vi "Fire DAQAcqModeChanged Event_DAQ.vi"(8 "error in (no error)":errorcluster, 10 "DAQState":variant, 11 "DAQ_Engine in":refnum<class "DAQ_Engine.lvclass">) -> (0 "error out":errorcluster, 3 "DAQ_Engine out":refnum<class "DAQ_Engine.lvclass">)   [LabVIEW 2019, in "DAQ_Engine.lvclass"]
doc: "Developed by Kevin Thompson\nkevin@thompsonengineering.net\n\nCopyright 2018-2020\nThompson Engineering, LLC"
uses:
  DAQ_Engine.lvclass
  Common/DataTypes/Acquisition Mode--cluster.ctl
  DataTypes/DAQAcqModeChg EvData--cluster.ctl
  DAQ_Engine.lvclass/DAQ_Engine.ctl
  Accessors/Get PublicEvents.vi
  Accessors/Get InverterDataAcqMode.vi
  Accessors/Set InverterDataAcqMode.vi
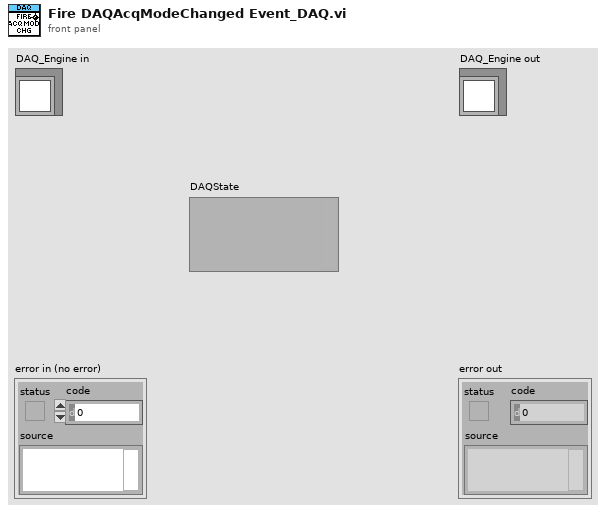
[diagram p1: front panel]
types:
  T1 = typedef "Acquisition Mode--cluster.ctl" = enum16{"3phase", "Single"}
  T2 = typedef "DAQ_Engine.lvclass/DAQAcqModeChg EvData--cluster.ctl" = cluster{"Time Stamp":timestamp, "OLD AcqMode":T1, "NEW AcqMode":T1}
  T3 = typedef "DAQ_Engine.lvclass/Public Events--cluster.ctl" = cluster{"DAQ_Engine.AsyncCmd Event":refnum<user-event>, "DAQ_Engine.AsyncMsg Event":refnum<user-event>, "stop process":refnum<user-event>, "DAQ_Engine.DAQStateChg Ev":refnum<user-event>, "DAQ_Engine.MeasSettingsChg Ev":refnum<user-event>, "DAQ_Engine.AcqModeChg Ev":refnum<user-event>}
  T4 = typedef "Type Descriptor Enumeration__ogtk.ctl" = enum8{"<Null>", "I8", "I16", "I32", "I64", "U8", "U16", "U32", "U64", "SGL", "DBL", "EXT", "CSG", "CDB", "CXT", "0x0F", "0x10", "0x11", "0x12", "0x13", "0x14", "Enum U8", "Enum U16", "Enum U32", "Enum U64", "SGL PQ", "DBL PQ", "EXT PQ", "CSG PQ", "CDB PQ", "CXT PQ", "0x1F", "0x20", "Boolean", "0x22", "0x23", "0x24", "0x25", "0x26", "0x27", "0x28", "0x29", "0x2A", "0x2B", "0x2C", "0x2D", "0x2E", "0x2F", "String", "0x31", "Path", "Pict", "0x34", "0x35", "0x36", "DAQ", "0x38", "0x39", "0x3A", "0x3B", "0x3C", "0x3D", "0x3E", "0x3F", "Array", "0x41", "0x42", "0x43", "0x44", "0x45", "0x46", "0x47", "0x48", "0x49", "0x4A", "0x4B", "0x4C", "0x4D", "0x4E", "0x4F", "Cluster", "0x51", "0x52", "Variant", "Waveform", "0x55", "0x56", "0x57", "0x58", "0x59", "0x5A", "0x5B", "0x5C", "0x5D", "0x5E", "0x5F", "0x60", "0x61", "0x62", "0x63", "0x64", "0x65", "0x66", "0x67", "0x68", "0x69", "0x6A", "0x6B", "0x6C", "0x6D", "0x6E", "0x6F", "Refnum"}
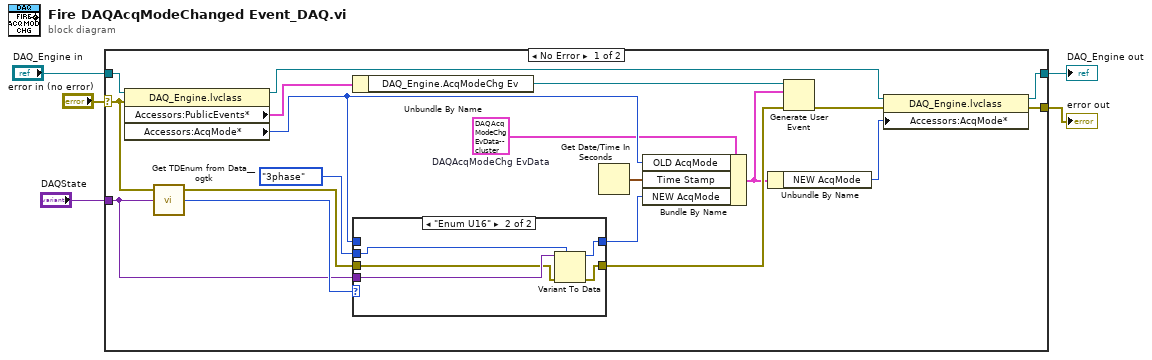
[diagram p0: block diagram]
diagram:
  n1 = case shown="No Error" "error in (no error)" {
    selector: "error in (no error)" -> [w12 w32]
    tunnel: [w13 w32] -> w4
    tunnel: [w17 w31] -> w2
    tunnel: "DAQ_Engine in" -> [w22 w31]
    tunnel: "DAQState" -> [w20 _]
    frame No Error {
      w6 = T2 {"Time Stamp"=timestamp(0 s since 1904-01-01), "OLD AcqMode"=enum."3phase", "NEW AcqMode"=enum."3phase"}  # DAQAcqModeChg EvData
      n2 = property class="DAQ_Engine.lvclass"(reference=w22, error in=w12) -> (reference out=w9:refnum<class "DAQ_Engine.lvclass">, "Accessors:PublicEvents*"=w10:T3, "Accessors:AcqMode*"=w7:T1)  [unwired: 1 out]
      n3 = call <userlib>:"Get TDEnum from Data__ogtk.vi"("Data"=w20) -> ("Type Descriptor Enumeration"=w21:T4)  [unwired: 4 in]
      n4 = Unbundle By Name(w10) -> ("DAQ_Engine.AcqModeChg Ev"=w11:refnum<user-event>)
      n5 = case shown="\"Enum U16\"" w21 {
        tunnel: w7 -> [w24 _]
        tunnel: w20 -> [_ w30]
        tunnel: [w24 w29] -> w19
        tunnel: Acquisition_Mode--cluster."3phase" ("Acquisition mode") -> [_ w28]
        tunnel: w12 -> [w25 w27]
        tunnel: [w25 w26] -> w18
        frame "<Null>", Default {
        }
        frame "Enum U16" {
          n6 = Variant To Data(error in=w27, type=w28, Variant=w30) -> (data=w29:T1, error out=w26:errorcluster)
        }
      }
      n7 = Get Date/Time In Seconds() -> (seconds since 1Jan1904=w23:timestamp)
      n8 = Bundle By Name(cluster=w6, "OLD AcqMode"=w7, "Time Stamp"=w23, "NEW AcqMode"=w19) -> (w16:T2)
      n9 = Unbundle By Name(w16) -> ("NEW AcqMode"=w15:T1)
      n10 = Generate User Event(user event=w11, event data cluster=w16, error in=w18) -> (error out=w14:errorcluster)  [unwired: 1 in, 1 out]
      n11 = property class="DAQ_Engine.lvclass"(reference=w9, error in=w14, "Accessors:AcqMode*"=w15) -> (reference out=w17:refnum<class "DAQ_Engine.lvclass">, error out=w13:errorcluster)
    }
    frame Error {
    }
  }
  "error out" <- w4
  "DAQ_Engine out" <- w2
